vi "Write to System Log.vi"(8 "error in (no error)":errorcluster, 10 "severity":i32(ring) caption="severity (Error)" items=["Error", "Warning", "Informational"], 11 "message":string) -> (0 "error out":errorcluster)   [LabVIEW 2020, in "NI_SystemLogging.lvlib"]
doc: "Writes a message to the nierrlog system log for storage and subsequent viewing."
uses:
  <vilib>/Utility/SystemLogging/NI_SystemLogging.lvlib
  systemLogging.dll
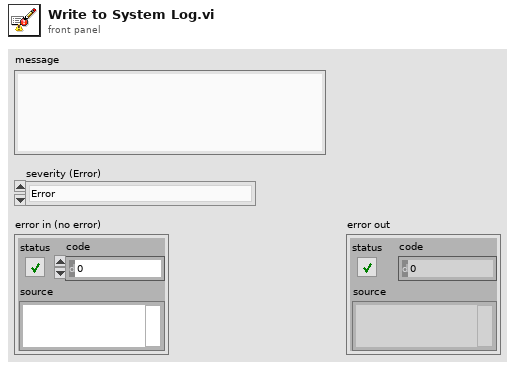
[diagram p1: front panel]
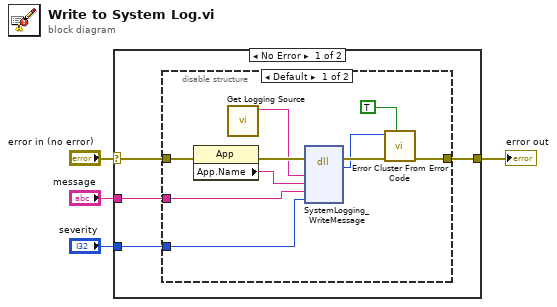
[diagram p0: block diagram]
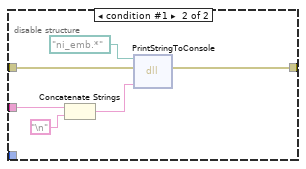
[diagram p2: hidden frame]
diagram:
  n1 = case shown="No Error" "error in (no error)" {
    selector: "error in (no error)" -> [w8 w25]
    tunnel: [w5 w25] -> w3
    tunnel: "severity" -> [w6 _]
    tunnel: "message" -> [w7 _]
    frame No Error {
      n2 = disable-structure shown="Default" {
        disable-tunnel: w8 -> [w18 w20]
        disable-tunnel: w7 -> [w16 w24]
        disable-tunnel: w6 -> [w15 _]
        disable-tunnel: [w14 w21] -> w5
        frame condition #0 (active) {
          n3 = property class="App"(error in=w18) -> (error out=w11:errorcluster, "App.Name"=w10:string)  [unwired: 1 in, 1 out]
          n4 = call <vilib>:"Get Logging Source.vi"() -> ("Logging Source"=w9:string)  [unwired: 11 in]
          n5 = dll-call lib="systemLogging.*" fn="SystemLogging_WriteMessage"(error in=w11, "source"=w9, "appName"=w10, "message"=w16, "severity"=w15) -> (error out=w17:errorcluster, "return type"=w13:i32)  [unwired: 6 in, 1 out]
          n6 = call <vilib>:"Error Cluster From Error Code.vi"("show call chain? (False)"=TRUE, "error in (no error)"=w17, "error code (0)"=w13) -> ("error out"=w14:errorcluster)  [unwired: 6 in]
        }
        frame condition #1 {
          n7 = Concatenate Strings(w24, "\n") -> (w22:string)
          n8 = dll-call lib="C:/Program Files (x86)/National Instruments/LabVIEW 2013/vi.lib/ni_emb.*" fn="PrintStringToConsole"(path in=path "ni_emb.*", error in=w20, "str"=w22) -> (error out=w21:errorcluster)  [unwired: 2 in, 2 out]
        }
      }
    }
    frame Error {
    }
  }
  "error out" <- w3
